vi "Geometric Matching with Calibration.vi"() -> ()   [LabVIEW 2014]
doc: "This example demonstrates how to calibrate an image to perform accurate geometric matching without correcting the image. First, the template pattern is learned. Then, test images and their associated calibration grids are loaded, the calibration is applied to the test image, and the template is found in the test image."
uses:
  <vilib>/vision/Pattern Matching.llb/IMAQ Match Range Setting.ctl
  <vilib>/vision/NI_Vision_Development_Module.lvlib
panel:
  out "Template":T1(plugin-control)
  out "Number of Matches Found":i32
  in  "Stop":bool
  in  "Delay (s.)":dbl(slide)=0.496 scale=0.0..2.0
  out "Image":T1(plugin-control)
  # "Overview: Demonstrates how to use geometric matching to locate parts in an image.\nRequirements: NI Vision Development Module\nInstructions: Run the VI."
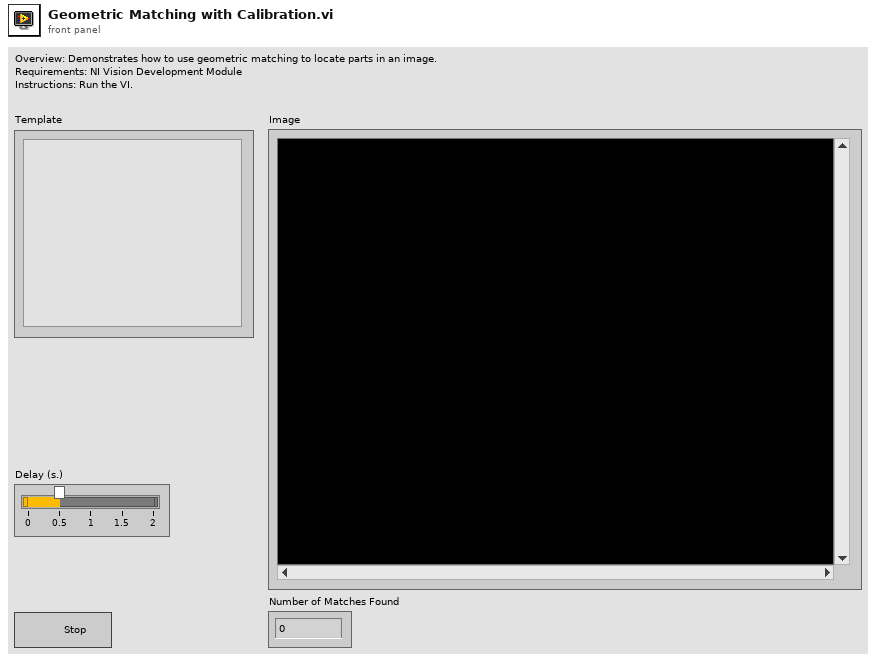
[diagram p1: front panel]
types:
  T1 = typedef "IMAQ Image.ctl" = refnum<image>
  T2 = cluster{"Setup Data Item":u16, "Item Value":dbl}[]
  T3 = typedef "IMAQ Match Range Setting.ctl" = cluster{"Match Constraints":u32, "Min":dbl, "Max":dbl}
  T4 = cluster{"Rotation":bool, "Scale":bool, "Occlusion":bool, "Reserved":bool, "Reserved":bool, "Reserved":bool}
  T5 = typedef "Image Type" = u32
  T6 = typedef "IMAQ GM Match Report.ctl" = cluster{"Position":cluster{"x":sgl, "y":sgl}, "Angle":sgl, "Scale":sgl, "Score":sgl, "Bounding Box":cluster{"x":sgl, "y":sgl}[], "Contrast Reversed":bool, "Occlusion %":sgl, "Template Target Curve Score":sgl, "Target Template Curve Score":sgl, "Correlation Score":sgl}
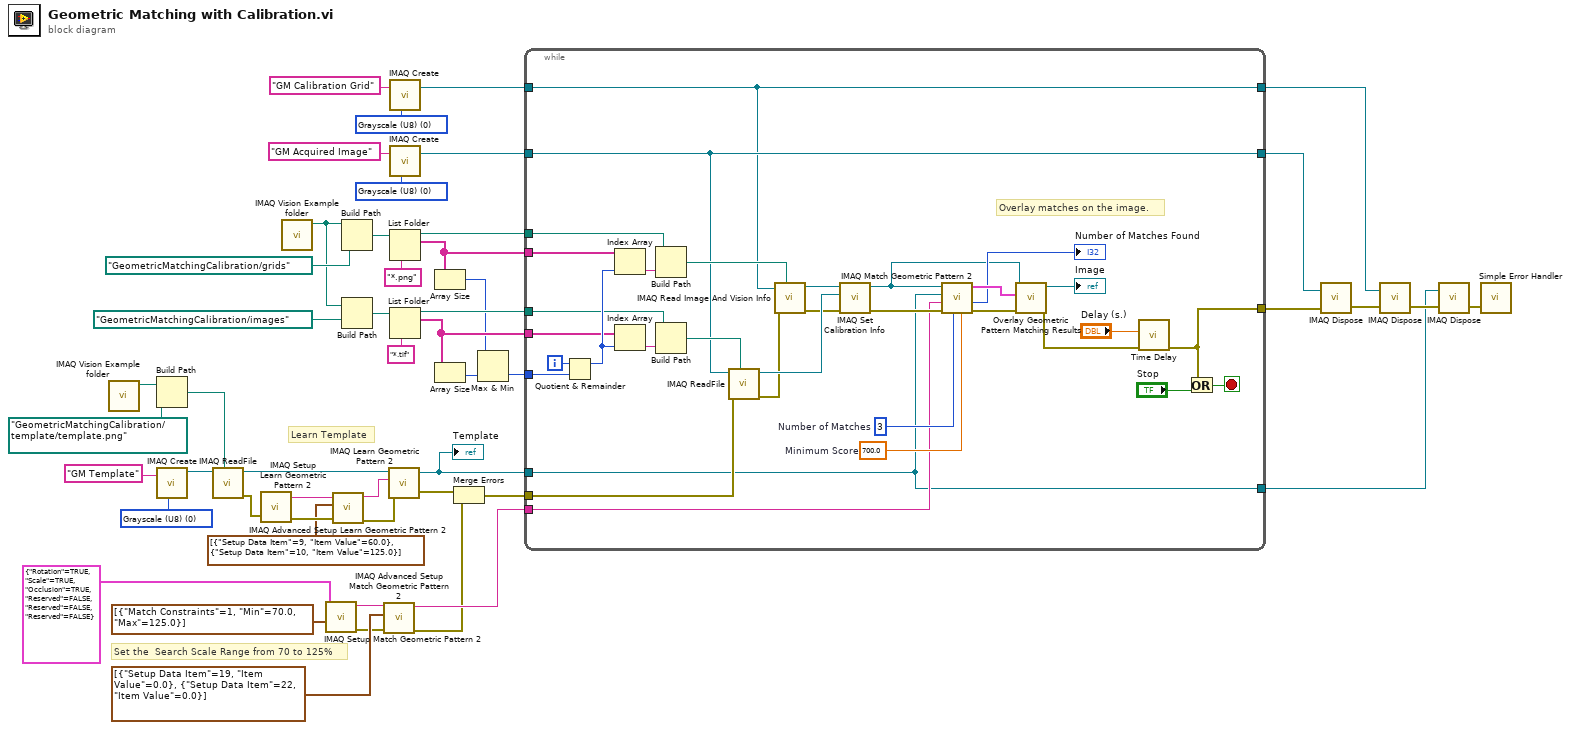
[diagram p0: block diagram]
diagram:
  w19 = T5 0 items=["Grayscale (U8)", "Grayscale (I16)", "Grayscale (SGL)", "Complex (CSG)", "RGB (U32)", "HSL (U32)", "RGB (U64)"] ("Image Type")
  w20 = T5 0 items=["Grayscale (U8)", "Grayscale (I16)", "Grayscale (SGL)", "Complex (CSG)", "RGB (U32)", "HSL (U32)", "RGB (U64)"] ("Image Type")
  w47 = T5 0 items=["Grayscale (U8)", "Grayscale (I16)", "Grayscale (SGL)", "Complex (CSG)", "RGB (U32)", "HSL (U32)", "RGB (U64)"] ("Image Type")
  # "Set the  Search Scale Range from 70 to 125%"
  # "Learn Template"
  n1 = call "IMAQ Vision Example folder.vi"() -> ("Example Image Path"=w45:path)  [unwired: 11 in]
  n2 = Build Path(base path=w45, name or relative path=path "GeometricMatchingCalibration/template/template.png") -> (appended path=w35:path)
  n3 = call "IMAQ Create"("Image Name"="GM Template", "Image Type"=w47) -> ("New Image"=w37:T1)  [unwired: 2 in, 2 out]
  n4 = call "IMAQ ReadFile"("File Path"=w35, "Image"=w37) -> ("error out"=w43:errorcluster, "Image Out"=w39:T1)  [unwired: 5 in, 3 out]
  n5 = call "IMAQ Setup Learn Geometric Pattern 2"("error in (no error)"=w43) -> ("error out"=w41:errorcluster, "Learn Geometric Pattern 2 Setup Data"=w42:string)  [unwired: 1 in]
  n6 = call "IMAQ Vision Example folder.vi"() -> ("Example Image Path"=w5:path)  [unwired: 11 in]
  n7 = call "IMAQ Setup Match Geometric Pattern 2"("Range Settings"=T3[] [{"Match Constraints"=1, "Min"=70.0, "Max"=125.0}], "Match Mode"=T4 {"Rotation"=TRUE, "Scale"=TRUE, "Occlusion"=TRUE, "Reserved"=FALSE, "Reserved"=FALSE, "Reserved"=FALSE}) -> ("error out"=w4:errorcluster, "Match Geometric Pattern 2 Setup Data"=w15:string)  [unwired: 8 in]
  n8 = call "IMAQ Advanced Setup Learn Geometric Pattern 2"("Learn Geometric Pattern 2 Setup Data In"=w42, "Advanced Geometric Learn Options 2"=T2 [{"Setup Data Item"=9, "Item Value"=60.0}, {"Setup Data Item"=10, "Item Value"=125.0}], "error in (no error)"=w41) -> ("Learn Geometric Pattern 2 Setup Data Out"=w38:string, "error out"=w40:errorcluster)  [unwired: 6 in]
  n9 = Build Path(base path=w5, name or relative path=path "GeometricMatchingCalibration/grids") -> (appended path=w33:path)
  n10 = Build Path(base path=w5, name or relative path=path "GeometricMatchingCalibration/images") -> (appended path=w32:path)
  n11 = call "IMAQ Advanced Setup Match Geometric Pattern 2"("Match Geometric Pattern 2 Setup Data In"=w15, "Advanced Geometric Match Options 2"=T2 [{"Setup Data Item"=19, "Item Value"=0.0}, {"Setup Data Item"=22, "Item Value"=0.0}], "error in (no error)"=w4) -> ("Match Geometric Pattern 2 Setup Data Out"=w12:string, "error out"=w2:errorcluster)  [unwired: 6 in]
  n12 = call "IMAQ Learn Geometric Pattern 2"("error in (no error)"=w40, "Learn Geometric Pattern 2 Setup Data"=w38, "Template Image"=w39) -> ("error out"=w3:errorcluster, "Template Image Out"=w11:T1)  [unwired: 7 in]
  "Template" <- w11
  n13 = call "IMAQ Create"("Image Name"="GM Calibration Grid", "Image Type"=w19) -> ("New Image"=w17:T1)  [unwired: 2 in, 2 out]
  n14 = call "IMAQ Create"("Image Name"="GM Acquired Image", "Image Type"=w20) -> ("New Image"=w22:T1)  [unwired: 2 in, 2 out]
  n15 = List Folder(path=w33, pattern="*.png") -> (path out=w29:path, filenames=w27:string[])  [unwired: 2 in, 2 out]
  n16 = List Folder(path=w32, pattern="*.tif") -> (path out=w28:path, filenames=w26:string[])  [unwired: 2 in, 2 out]
  n17 = Array Size(array=w27) -> (size(s)=w24:i32)
  n18 = Array Size(array=w26) -> (size(s)=w25:i32)
  n19 = Merge Errors(w3, w2) -> (w1:errorcluster)
  n20 = Max & Min(x=w24, y=w25) -> (min(x,y)=w23:i32)  [unwired: 1 out]
  n21 = while {
    tunnel: [w82] -> w49
    tunnel: w11 -> [w52]
    tunnel: w29 -> [w65]
    tunnel: w27 -> [w68]
    tunnel: w28 -> [w64]
    tunnel: w26 -> [w67]
    tunnel: w23 -> [w57]
    tunnel: w22 -> [w53]
    tunnel: w17 -> [w51]
    tunnel: w12 -> [w56]
    tunnel: w1 -> [w55]
    tunnel: [w52] -> w8
    tunnel: [w53] -> w7
    tunnel: [w51] -> w6
    i -> [w58]
    stop <- w83 stop-if-true
    w79 = sgl 700.0  # Minimum Score
    w81 = 3  # Number of Matches
    # "Overlay matches on the image."
    n22 = Quotient & Remainder(x=w58, y=w57) -> (x-y*floor(x/y)=w69:i32)  [unwired: 1 out]
    n23 = Index Array(array=w68, index=w69) -> (element=w66:string)
    n24 = Index Array(array=w67, index=w69) -> (element=w63:string)
    n25 = Build Path(base path=w65, name or relative path=w66) -> (appended path=w61:path)
    n26 = Build Path(base path=w64, name or relative path=w63) -> (appended path=w62:path)
    n27 = call "IMAQ ReadFile"("File Path"=w62, "error in (no error)"=w55, "Image"=w53) -> ("error out"=w59:errorcluster, "Image Out"=w74:T1)  [unwired: 4 in, 3 out]
    n28 = call "IMAQ Read Image And Vision Info"("File Path"=w61, "error in (no error)"=w59, "Image"=w51) -> ("error out"=w60:errorcluster, "Image Out"=w73:T1)  [unwired: 6 in, 1 out]
    n29 = call "IMAQ Set Calibration Info"("error in (no error)"=w60, "Image Dst"=w74, "Image Src"=w73) -> ("error out"=w71:errorcluster, "Calibrated Image"=w72:T1)  [unwired: 7 in]
    n30 = call "IMAQ Match Geometric Pattern 2"("Minimum Match Score"=w79, "Number of Matches Requested"=w81, "error in (no error)"=w71, "Match Geometric Pattern 2 Setup Data"=w56, "Template Image"=w52, "Image"=w72) -> ("error out"=w78:errorcluster, "Number of Matches"=→"Number of Matches Found":i32, "Matches (pixel)"=w80:T6[])  [unwired: 1 in, 2 out]
    n31 = call "Overlay Geometric Pattern Matching Results.vi"("error in"=w78, "Matches"=w80, "Image"=w72) -> ("error out"=w76:errorcluster, "Image Out"=→"Image":T1)  [unwired: 2 in, 5 out]
    n32 = call "Time Delay"("error in (no error)"=w76, "Delay Time (s)"="Delay (s.)") -> ("error out"=w82:errorcluster)  [unwired: 9 in]
    n33 = Or(x=w82, y="Stop") -> (x .or. y?=w83:bool)
  }
  n34 = call "IMAQ Dispose"("Image"=w7, "error in (no error)"=w49) -> ("error out"=w44:errorcluster)  [unwired: 1 in, 3 out]
  n35 = call "IMAQ Dispose"("Image"=w6, "error in (no error)"=w44) -> ("error out"=w10:errorcluster)  [unwired: 1 in, 3 out]
  n36 = call "IMAQ Dispose"("Image"=w8, "error in (no error)"=w10) -> ("error out"=w9:errorcluster)  [unwired: 1 in, 3 out]
  n37 = call <vilib>:"Simple Error Handler.vi"("error in (no error)"=w9) -> ()  [unwired: 4 in, 5 out]
